vi "SPI Get Channel Info.vi"(8 "error in (no error)":errorcluster, 11 "index":u32) -> (0 "error out":errorcluster, 1 "Flags":u32 format="%b", 2 "Description":string, 3 "Serial number":string, 4 "Type":u32, 5 "ftHandle":u32 format="%08x", 6 "ID":u32 format="%08x", 7 "LocId":u32)   [LabVIEW 2016, in "libMPSSE-SPI.lvlib"]
doc: "FTDI_API FT_STATUS SPI_GetChannelInfo(uint32 index,\n FT_DEVICE_LIST_INFO_NODE *chanInfo);"
uses:
  libMPSSE-SPI.lvlib
  libMPSSE.dll
panel:
  out "function return":u32
  # "The flag value is a 4-byte bit map containing miscellaneous data as defined Appendix A – Type\nDefinitions. \n  Bit 0 (least significant bit) of this number indicates if the port is open (1) or closed (0). \n  Bit 1 indicates if the device is enumerated as a high-speed USB device (2) or a full-speed USB device (0). \n  The remaining bits (2 - 31) are reserved."
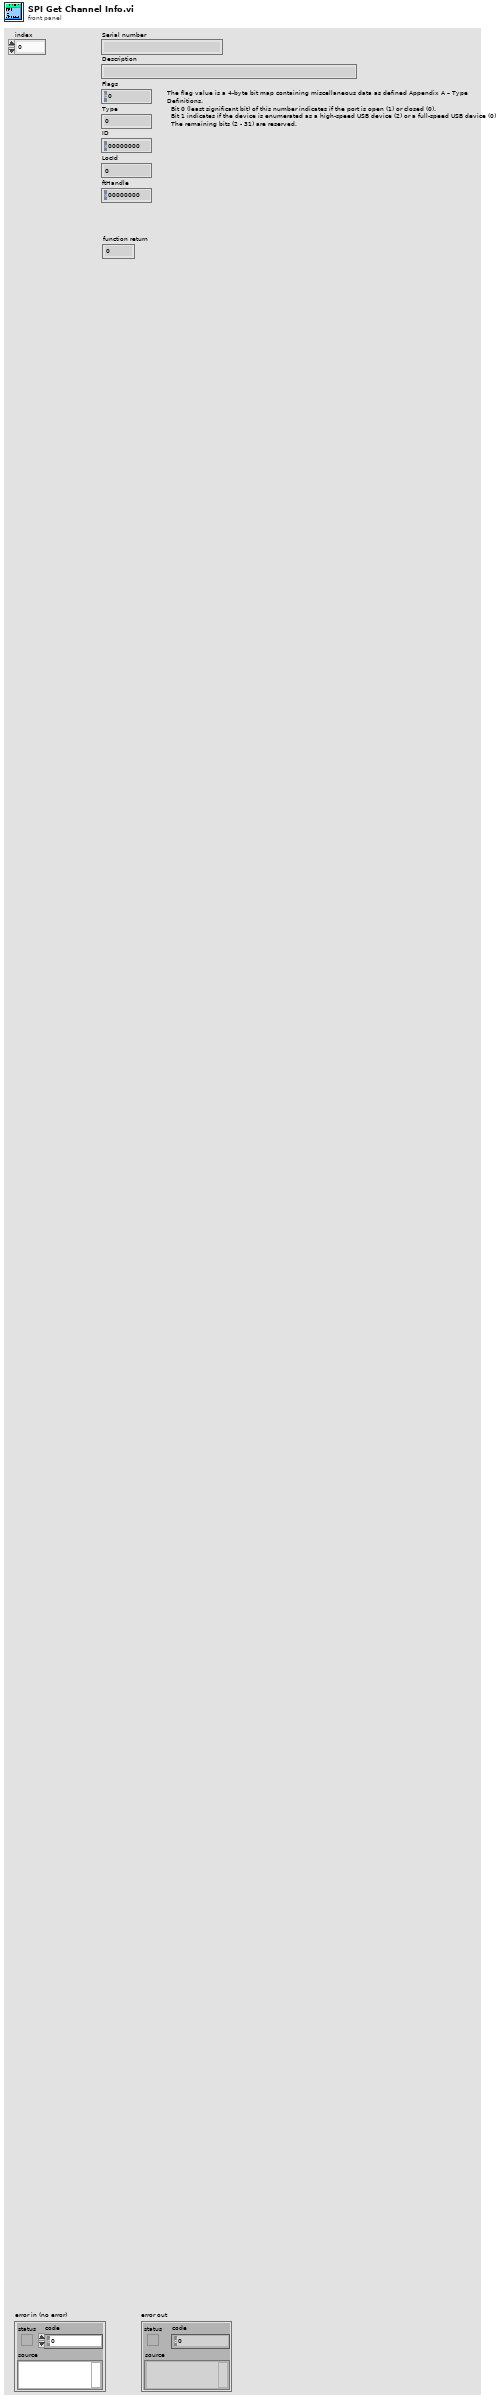
[diagram p1: front panel]
types:
  T1 = cluster{"Flags":u32, "Type":u32, "ID":u32, "LocId":u32, "SerialNumber[0]":i8, "SerialNumber[1]":i8, "SerialNumber[2]":i8, "SerialNumber[3]":i8, "SerialNumber[4]":i8, "SerialNumber[5]":i8, "SerialNumber[6]":i8, "SerialNumber[7]":i8, "SerialNumber[8]":i8, "SerialNumber[9]":i8, "SerialNumber[10]":i8, "SerialNumber[11]":i8, "SerialNumber[12]":i8, "SerialNumber[13]":i8, "SerialNumber[14]":i8, "SerialNumber[15]":i8, "Description[0]":i8, "Description[1]":i8, "Description[2]":i8, "Description[3]":i8, "Description[4]":i8, "Description[5]":i8, "Description[6]":i8, "Description[7]":i8, "Description[8]":i8, "Description[9]":i8, "Description[10]":i8, "Description[11]":i8, "Description[12]":i8, "Description[13]":i8, "Description[14]":i8, "Description[15]":i8, "Description[16]":i8, "Description[17]":i8, "Description[18]":i8, "Description[19]":i8, "Description[20]":i8, "Description[21]":i8, "Description[22]":i8, "Description[23]":i8, "Description[24]":i8, "Description[25]":i8, "Description[26]":i8, "Description[27]":i8, "Description[28]":i8, "Description[29]":i8, "Description[30]":i8, "Description[31]":i8, "Description[32]":i8, "Description[33]":i8, "Description[34]":i8, "Description[35]":i8, "Description[36]":i8, "Description[37]":i8, "Description[38]":i8, "Description[39]":i8, "Description[40]":i8, "Description[41]":i8, "Description[42]":i8, "Description[43]":i8, "Description[44]":i8, "Description[45]":i8, "Description[46]":i8, "Description[47]":i8, "Description[48]":i8, "Description[49]":i8, "Description[50]":i8, "Description[51]":i8, "Description[52]":i8, "Description[53]":i8, "Description[54]":i8, "Description[55]":i8, "Description[56]":i8, "Description[57]":i8, "Description[58]":i8, "Description[59]":i8, "Description[60]":i8, "Description[61]":i8, "Description[62]":i8, "Description[63]":i8, "ftHandle":u32}
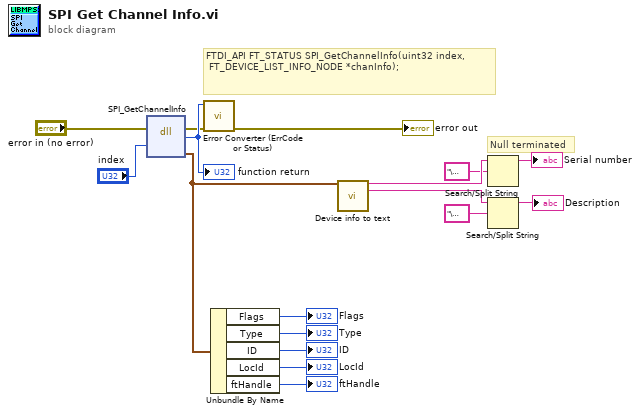
[diagram p0: block diagram]
diagram:
  # "Null terminated"
  # "FTDI_API FT_STATUS SPI_GetChannelInfo(uint32 index,\n\tFT_DEVICE_LIST_INFO_NODE *chanInfo);"
  n1 = dll-call lib="C:/Users/inca/Desktop/FTDI/libMPSSE-SPI LabVIEW/libMPSSE.*" fn="SPI_GetChannelInfo"(error in="error in (no error)", "index"="index") -> (error out=w14:errorcluster, w17:u32, "chanInfo out"=w8:T1)  [unwired: 4 in, 1 out]
  "function return" <- w17
  n2 = call "Error Converter (ErrCode or Status).vi"("error in (no error)"=w14, "error code"=w17) -> ("error out"=→"error out":errorcluster)  [unwired: 9 in]
  n3 = Unbundle By Name(w8) -> ("Flags"=→"Flags":u32, "Type"=→"Type":u32, "ID"=→"ID":u32, "LocId"=→"LocId":u32, "ftHandle"=→"ftHandle":u32)
  n4 = call "Device info to text.vi"("chanInfo out"=w8) -> ("Serial number"=w6:string, "Description"=w1:string)  [unwired: 13 in]
  n5 = Search/Split String(string=w6, search string/char (-)="\u0000") -> (substring before match=→"Serial number":string)  [unwired: 1 in, 2 out]
  n6 = Search/Split String(string=w1, search string/char (-)="\u0000") -> (substring before match=→"Description":string)  [unwired: 1 in, 2 out]
